vi "MPDSnC Engine.vi"(0 "Notifier Name":string, 11 "COM Port":string[](array[string])) -> ()   [LabVIEW 2016]
uses:
  AOTF Controls/AOTF Lines Lines Control.ctl
  AOTF Controls/AOTF Notifier Element.ctl
  AOTF Controls/AOTF Actions.ctl
  <vilib>/Instr/_visa.llb/VISA Configure Serial Port (Instr).vi
panel:
  in  "Line On/Off":bool
  in  "Laser Wavelength (nm)":string
  out "Write Response":string
  in  "Blank":bool
  in  "Quit":bool
  in  "Power":dbl(slide) scale=0.0..100.0
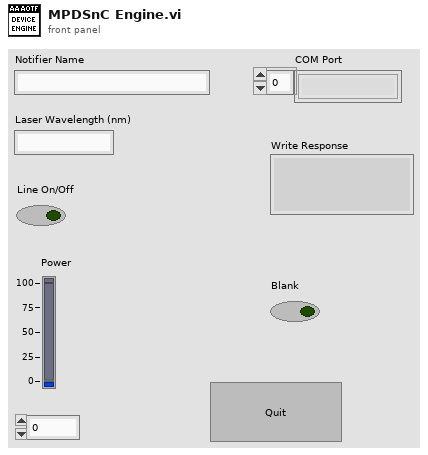
[diagram p1: front panel]
types:
  T1 = typedef "AOTF Notifier Element.ctl" = cluster{"AOTF Action":T2, "Laser Line":string, "Power (%)":dbl, "Beam Blank On/Off":bool, "Line On/Off":bool, "Error":errorcluster}
  T2 = typedef "AOTF Actions.ctl" = enum16{"Error Check", "Blank", "Line On/Off", "Set Power", "Status", "Quit"}
  T3 = typedef "AOTF Lines Lines Control.ctl" = cluster{"Wavelength":u16[], "AO Line":string[]}
  T4 = enum32{"Invalid", "Standard", "Closed", "Hidden", "Minimized", "Maximized"}
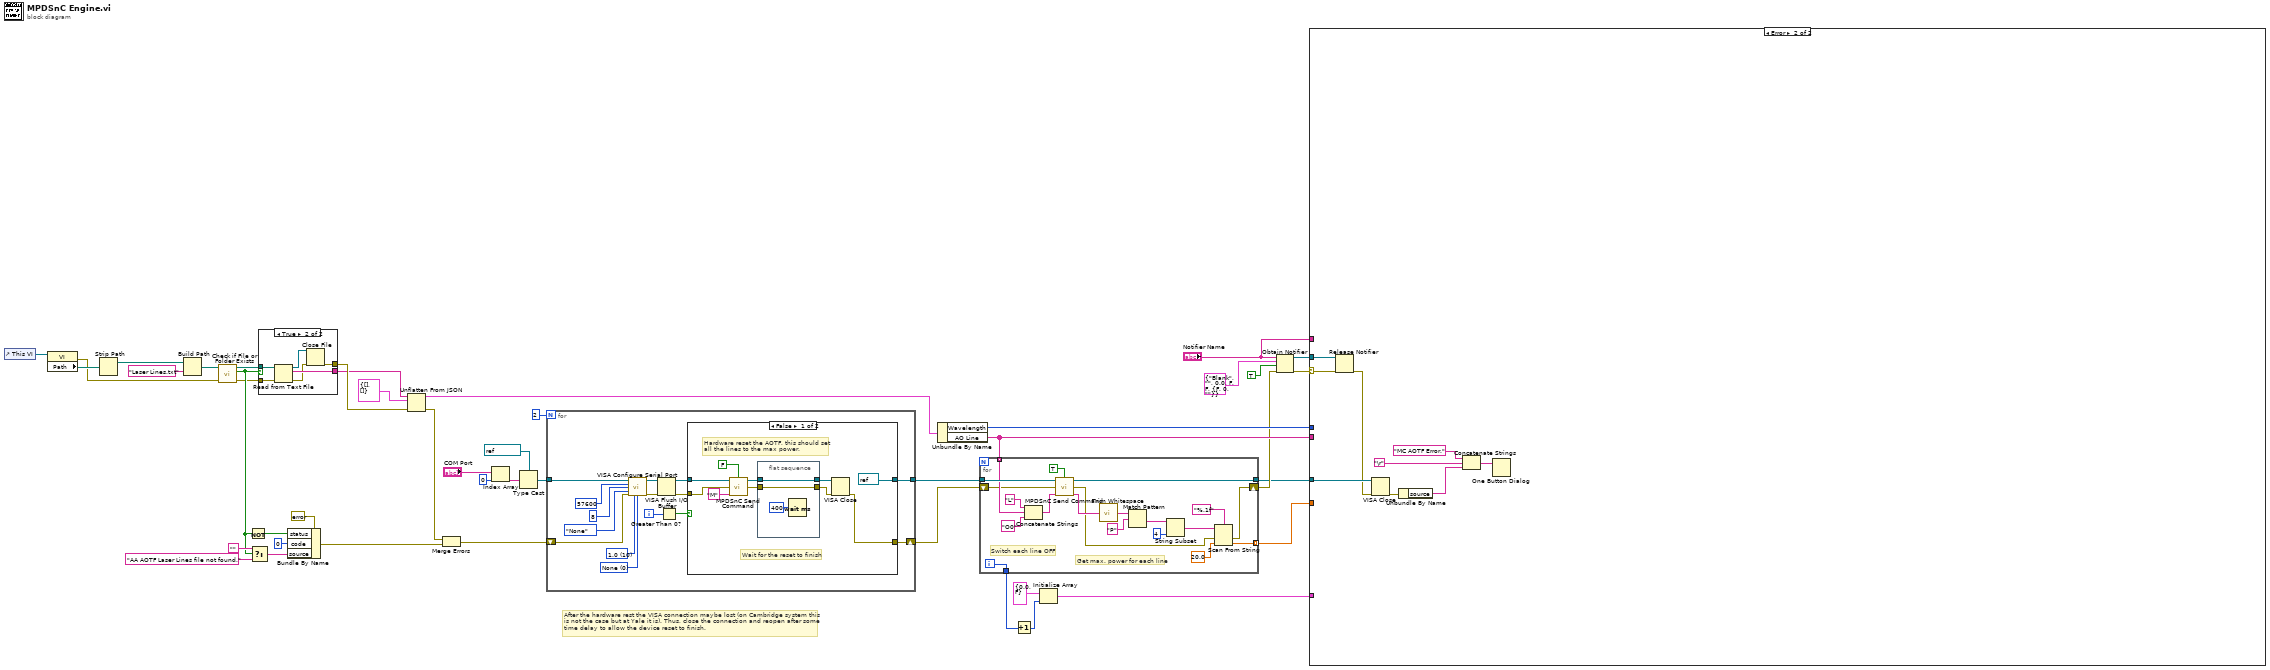
[diagram p0: block diagram]
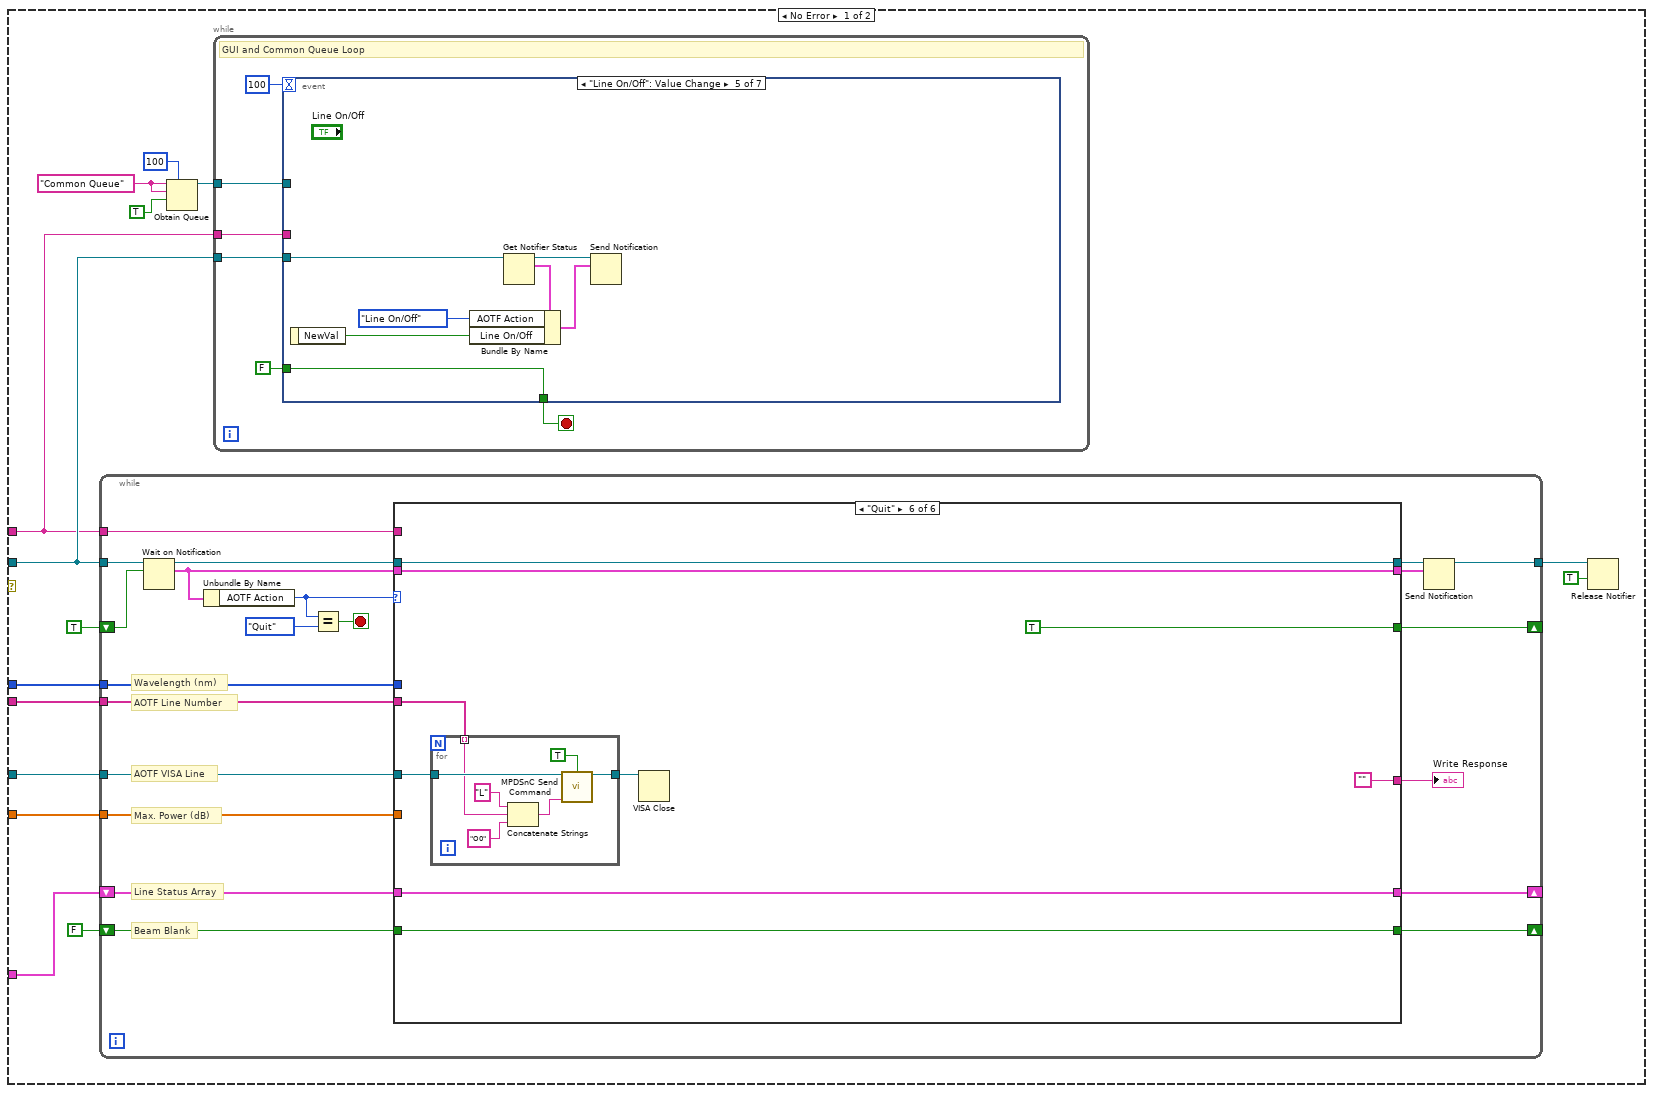
[diagram p3: hidden frame]
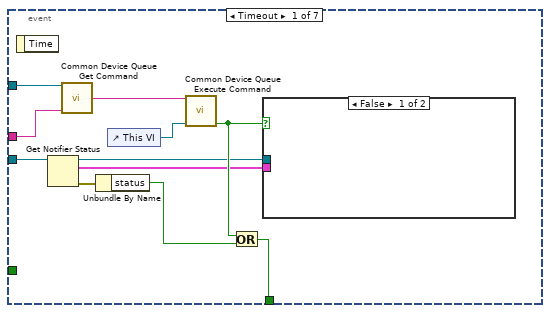
[diagram p4: hidden frame]
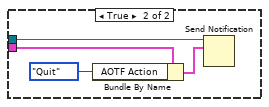
[diagram p5: hidden frame]
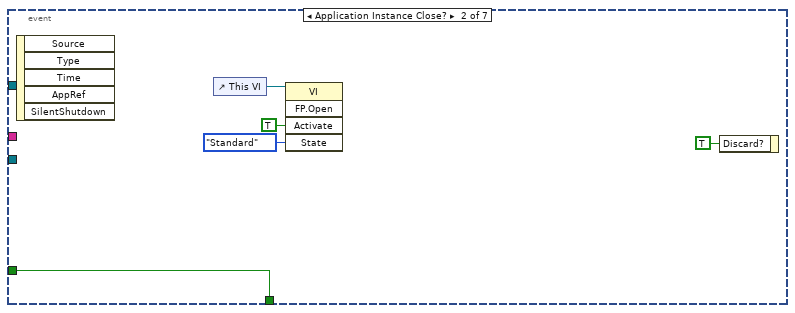
[diagram p6: hidden frame]
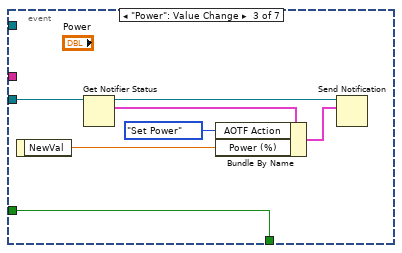
[diagram p7: hidden frame]
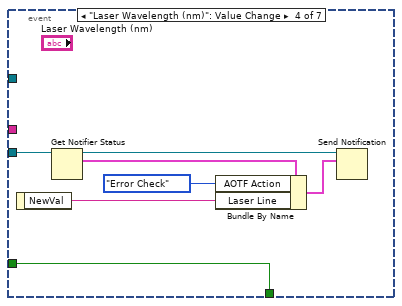
[diagram p8: hidden frame]
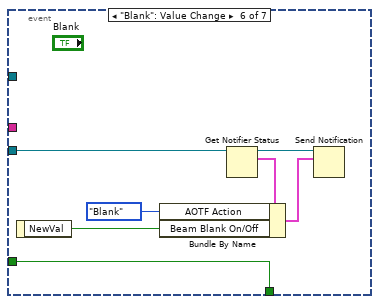
[diagram p9: hidden frame]
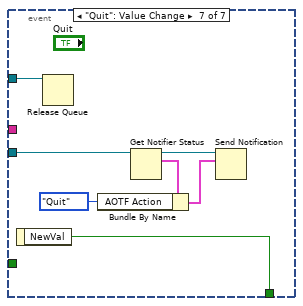
[diagram p10: hidden frame]
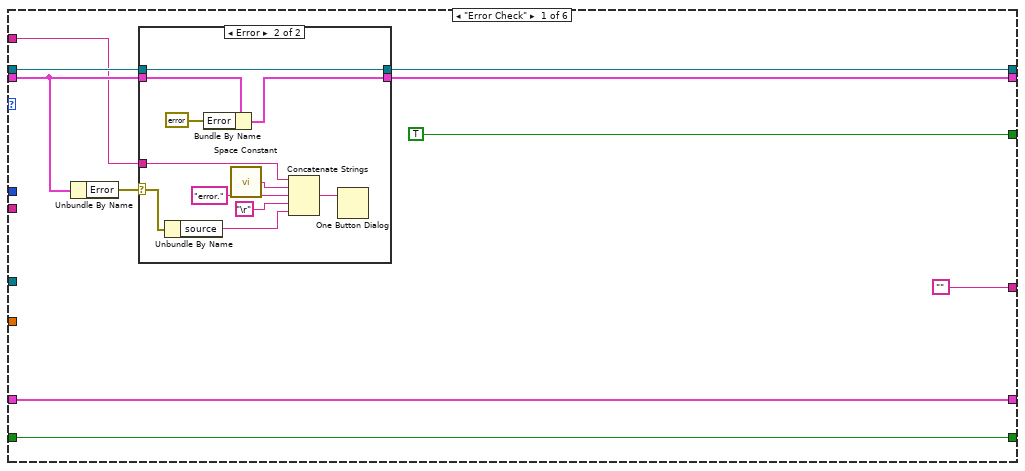
[diagram p11: hidden frame]
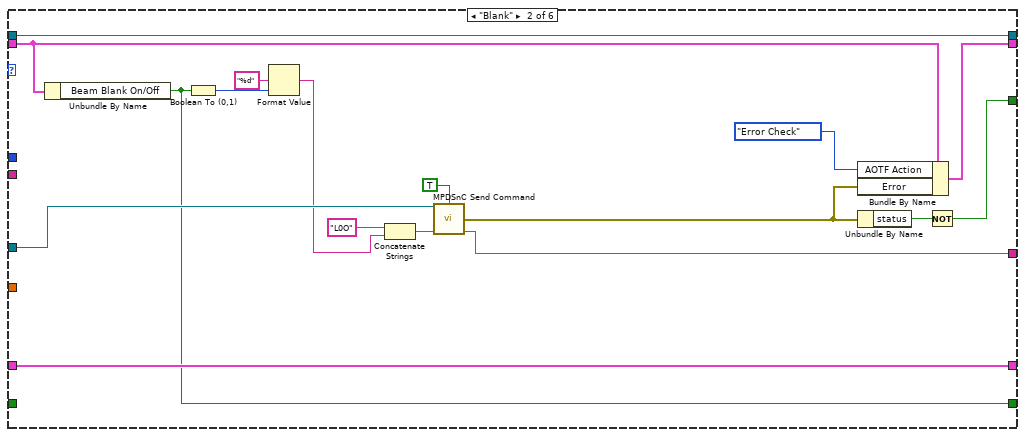
[diagram p13: hidden frame]
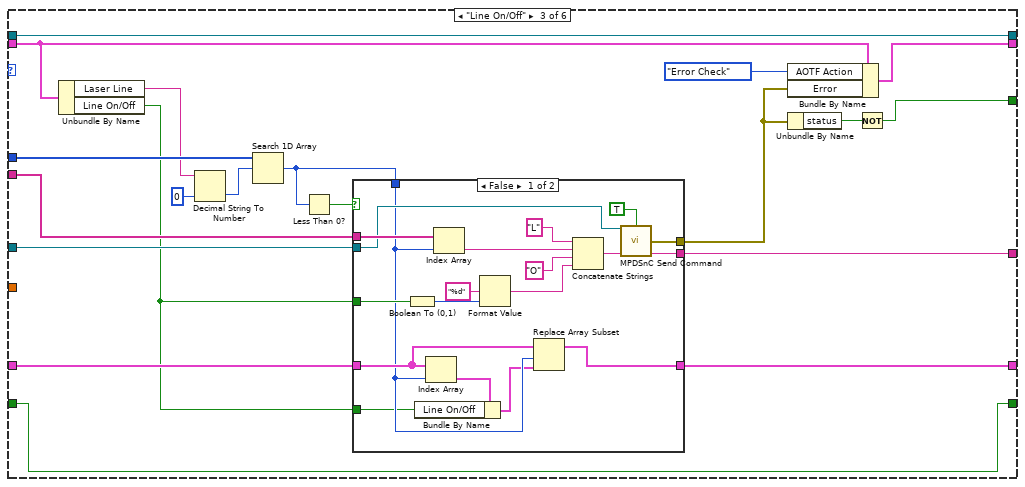
[diagram p14: hidden frame]
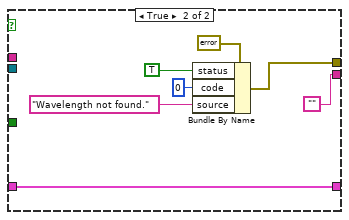
[diagram p15: hidden frame]
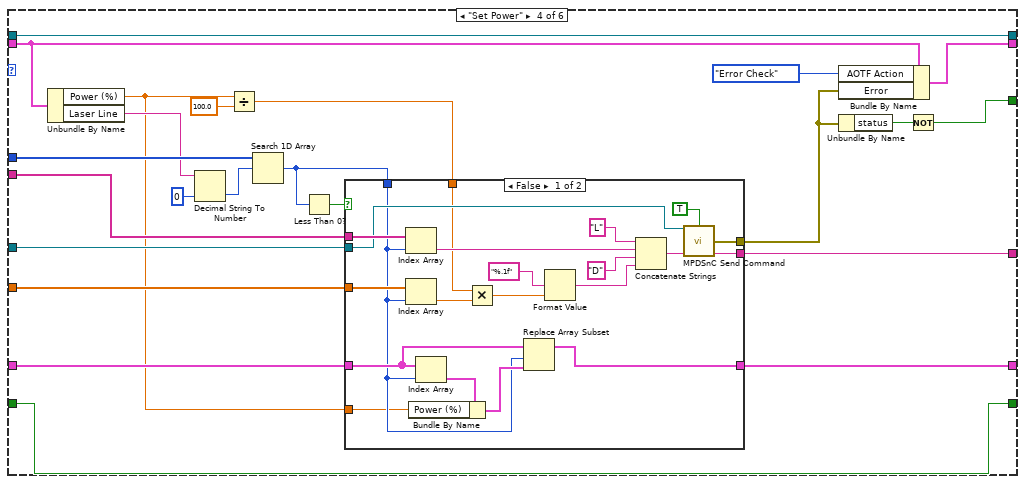
[diagram p16: hidden frame]
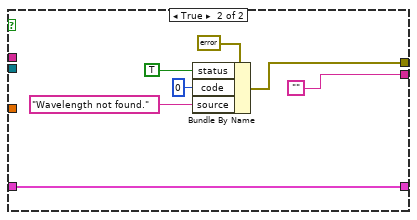
[diagram p17: hidden frame]
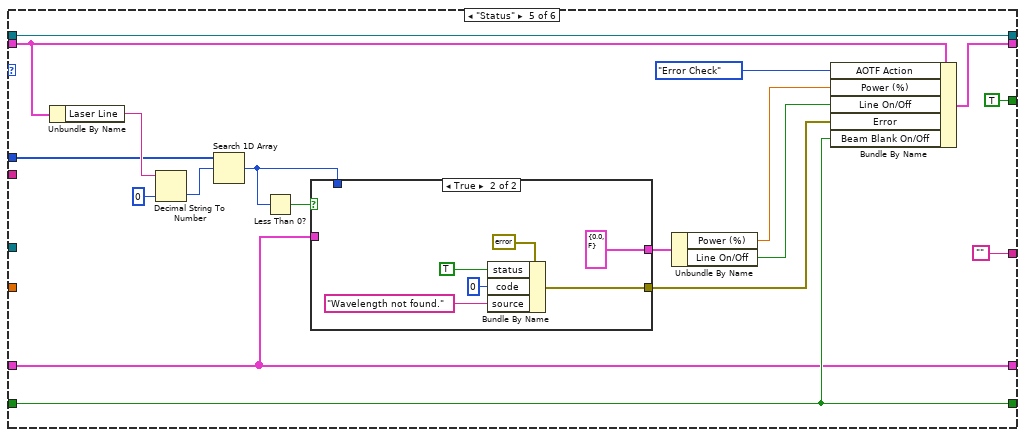
[diagram p18: hidden frame]
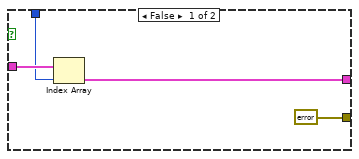
[diagram p19: hidden frame]
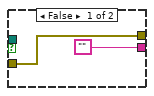
[diagram p20: hidden frame]
diagram:
  # "After the hardware rest the VISA connection maybe lost (on Cambridge system this\nis not the case but at Yale it is). Thus, close the connection and reopen after some\ntime delay to allow the device reset to finish."
  n1 = control-ref of="This VI"() -> (w44:refnum<vi>)
  n2 = property class="VI"(reference=w44) -> (error out=w31:errorcluster, "Path"=w43:path)  [unwired: 1 in, 1 out]
  n3 = Strip Path(path=w43) -> (stripped path=w42:path)  [unwired: 1 out]
  n4 = Build Path(base path=w42, name or relative path="Laser Lines.txt") -> (appended path=w40:path)
  n5 = call <vilib>:"Check if File or Folder Exists.vi"("error in (no error)"=w31, "path"=w40) -> ("error out"=w30:errorcluster, "file or folder exists?"=w33:bool, "dup path"=w32:path)  [unwired: 7 in]
  n6 = Not(x=w33) -> (.not. x?=w38:bool)
  n7 = Select(t="", s=w33, f="AA AOTF Laser Lines file not found." ("source")) -> (s? t:f=w34:string)
  n8 = case shown="True" w33 {
    tunnel: w32 -> [_ w52]
    tunnel: ["" w51] -> w26
    tunnel: w30 -> [w45 w49]
    tunnel: [w45 w47] -> w29
    frame False {
    }
    frame True {
      n9 = Read from Text File(file (use dialog)=w52, error in=w49) -> (refnum out=w50:refnum<file>, text=w51:string, error out=w48:errorcluster)  [unwired: 2 in, 1 out]
      n10 = Close File(refnum=w50, error in=w48) -> (error out=w47:errorcluster)  [unwired: 1 out]
    }
  }
  n11 = Bundle By Name(cluster=errorcluster {"status"=FALSE, "code"=0, "source"=""} ("Error"), "status"=w38, "code"=0, "source"=w34) -> (w27:errorcluster)
  n12 = Unflatten From JSON(JSON string=w26, type and defaults=T3 {"Wavelength"=[], "AO Line"=[]} ("Laser Lines"), error in (no error)=w29) -> (value=w24:T3, error out=w28:errorcluster)  [unwired: 4 in]
  n13 = Merge Errors(w28, w27) -> (w19:errorcluster)
  n14 = Index Array(array="COM Port", index=0) -> (element=w5:string)
  n15 = Type Cast(type=refnum<visa-resource-name> "COM6" ("reference"), x=w5) -> (*(type *) &x=w1:refnum<visa-resource-name>)
  n16 = for {
    N: 2 -> [_]
    tunnel: [w59] -> w21
    shift-right: [w57] -> w20
    shift-left: w19 -> [w56]
    tunnel: w1 -> [w53]
    i -> [w55]
    w67 = u16 0 items=["None", "XON/XOFF", "RTS/CTS", "XON/XOFF & RTS/CTS", "DTR/DSR", "XON/XOFF & DTR/DSR"] ("flow control (0:none)")
    w66 = u16 10 items=["1.0"=10, "1.5"=15, "2.0"=20] ("stop bits (10: 1 bit)")
    n17 = call-poly "VISA Configure Serial Port"("VISA resource name"=w53, "baud rate (9600)"=u32 57600, "data bits (8)"=u16 8, "parity (0:none)"=enum16{"None", "Odd", "Even", "Mark", "Space"}."None", "error in (no error)"=w56, "stop bits (10: 1 bit)"=w66, "flow control (0:none)"=w67) -> ("VISA resource name out"=w62:refnum<visa-resource-name>, "error out"=w61:errorcluster)  [unwired: 7 in]
    n18 = VISA Flush I/O Buffer(VISA resource name=w62, error in (no error)=w61) -> (VISA resource name out=w60:refnum<visa-resource-name>, error out=w58:errorcluster)  [unwired: 1 in]
    n19 = Greater Than 0?(x=w55) -> (x > 0?=w54:bool)
    n20 = case shown="False" w54 {
      tunnel: w60 -> [w77 w82]
      tunnel: [refnum<visa-resource-name> refnum ("VISA resource name") w82] -> w59
      tunnel: w58 -> [w76 w81]
      tunnel: [w69 w81] -> w57
      frame False {
        # "Wait for the reset to finish"
        # "Hardware reset the AOTF, this should set\nall the lines to the max power."
        n21 = call "MPDSnC Send Command.vi"("VISA Ref"=w77, "Wait for Reply?"=FALSE, "Error In"=w76, "Command"="M") -> ("VISA Ref Out"=w73:refnum<visa-resource-name>, "Error Out"=w72:errorcluster)  [unwired: 9 in, 1 out]
        n22 = flat-sequence {
          tunnel: [w80] -> w71
          tunnel: w73 -> [w80]
          tunnel: w72 -> [w78]
          tunnel: [w78] -> w70
          frame #0 {
            n23 = Wait (ms)(milliseconds to wait=u32 400) -> ()  [unwired: 1 out]
          }
        }
        n24 = VISA Close(VISA resource name=w71, error in (no error)=w70) -> (error out=w69:errorcluster)
      }
      frame True {
      }
    }
  }
  n25 = Unbundle By Name(w24) -> ("Wavelength"=w23:u16[], "AO Line"=w22:string[])
  n26 = for {
    tunnel: w21 -> [w101]
    tunnel: w22 -> [w99] mode=indexing
    tunnel: [w95] -> w11
    tunnel: [w88] -> w12 mode=indexing
    shift-right: [w84] -> w18
    shift-left: w20 -> [w86]
    tunnel: [w83] -> w9
    i -> [w83]
    # "Get max. power for each line"
    # "Switch each line OFF"
    n27 = Concatenate Strings("L", w99, "O0" ("string")) -> (w98:string)
    n28 = call "MPDSnC Send Command.vi"("VISA Ref"=w101, "Wait for Reply?"=TRUE, "Error In"=w86, "Command"=w98) -> ("VISA Ref Out"=w95:refnum<visa-resource-name>, "Error Out"=w85:errorcluster, "Response"=w96:string)  [unwired: 9 in]
    n29 = call <vilib>:"Trim Whitespace.vi"("string"=w96) -> ("trimmed string"=w94:string)  [unwired: 1 in]
    n30 = Match Pattern(string=w94, regular expression="P") -> (after substring=w92:string)  [unwired: 1 in, 3 out]
    n31 = String Subset(string=w92, length (rest)=4 ("length (rest)")) -> (substring=w90:string)  [unwired: 1 in]
    n32 = Scan From String(format string="%.1f", input string=w90, error in=w85, default 1=20.0 ("default value 1")) -> (error out=w84:errorcluster, output 1=w88:dbl)  [unwired: 1 in, 2 out]
  }
  n33 = Increment(x=w9) -> (x+1=w8:i32)
  n34 = Initialize Array(cluster{"Power (%)":dbl, "Line On/Off":bool} {"Power (%)"=0.0, "Line On/Off"=FALSE} ("Line Staus Cluster"), w8) -> (w7:cluster{"Power (%)":dbl, "Line On/Off":bool}[])
  n35 = Obtain Notifier(name (unnamed)="Notifier Name", notification data type=T1 {"AOTF Action"=enum."Blank", "Laser Line"="", "Power (%)"=0.0, "Beam Blank On/Off"=FALSE, "Line On/Off"=FALSE, "Error"={"status"=FALSE, "code"=0, "source"=""}} ("AOTFQueueCtrl"), create if not found? (T)=TRUE, error in (no error)=w18) -> (notifier out=w15:refnum<notifier>, error out=w14:errorcluster)  [unwired: 1 out]
  n36 = case shown="Error" w14 {
    selector: w14 -> [_ w388]
    tunnel: w15 -> [w113 w389]
    tunnel: "Notifier Name" -> [w109 _]
    tunnel: w23 -> [w108 _]
    tunnel: w22 -> [w107 _]
    tunnel: w12 -> [w106 _]
    tunnel: w11 -> [w105 w383]
    tunnel: w7 -> [w104 _]
    frame No Error {
      w117 = "Common Queue" ("Unique Notifier Name")
      n37 = while {
        tunnel: w113 -> [w199]
        shift-right: [w190] -> _
        shift-left: TRUE ("ignore previous (F)") -> [w198]
        tunnel: [w189] -> w111
        tunnel: w109 -> [w188]
        tunnel: w108 -> [w187]
        tunnel: w107 -> [w186]
        tunnel: w106 -> [w185]
        tunnel: w105 -> [w184]
        shift-right: [w179] -> _
        shift-left: w104 -> [w182]
        shift-right: [w180] -> _
        shift-left: FALSE -> [w181]
        stop <- w193 stop-if-true
        # "Wavelength (nm)"
        # "AOTF Line Number"
        # "Line Status Array"
        # "Beam Blank"
        # "AOTF VISA Line"
        # "Max. Power (dB)"
        n38 = Wait on Notification(notifier=w199, ignore previous (F)=w198) -> (notifier out=w197:refnum<notifier>, notification=w196:T1)  [unwired: 2 in, 2 out]
        n39 = Unbundle By Name(w196) -> ("AOTF Action"=w195:T2)
        n40 = Equal?(x=w195, y=AOTF_Actions."Quit") -> (x = y?=w193:bool)
        n41 = case shown="\"Quit\"" w195 {
          tunnel: w197 -> [w209 w239 w255 w308 w353 w373]
          tunnel: w196 -> [w207 w238 w257 w304 w348 w372]
          tunnel: [w205 w239 w255 w308 w353 w373] -> w192
          tunnel: [w204 w237 w256 w303 w344 w372] -> w191
          tunnel: [TRUE w234 w244 w302 TRUE TRUE] -> w190
          tunnel: w188 -> [w206 _ _ _ _ _]
          tunnel: w187 -> [_ _ w252 w299 w349 _]
          tunnel: w186 -> [_ _ w249 w295 _ w367]
          tunnel: w185 -> [_ _ _ w292 _ _]
          tunnel: w184 -> [_ w232 w248 w291 _ w366]
          tunnel: ["" w225 w246 w290 "" ""] -> w183
          tunnel: w182 -> [w201 w224 w243 w289 w337 w369]
          tunnel: w181 -> [w200 _ w241 w286 w338 w368]
          tunnel: [w200 w223 w241 w286 w338 w368] -> w180
          tunnel: [w201 w224 w242 w287 w337 w369] -> w179
          frame "Error Check" {
            n42 = Unbundle By Name(w207) -> ("Error"=w208:errorcluster)
            n43 = case shown="Error" w208 {
              selector: w208 -> [_ w215]
              tunnel: w207 -> [w210 w219]
              tunnel: [w211 w217] -> w205
              tunnel: w209 -> [w211 w217]
              tunnel: w206 -> [_ w214]
              tunnel: [w210 w216] -> w204
              frame No Error {
              }
              frame Error {
                n44 = Unbundle By Name(w215) -> ("source"=w213:string)
                n45 = Bundle By Name(cluster=w219, "Error"=errorcluster {"status"=FALSE, "code"=0, "source"=""}) -> (w216:T1)
                n46 = call <vilib>:"Space Constant.vi"() -> ("String"=w222:string)
                n47 = Concatenate Strings(w214, w222, "error." ("string"), "\r", w213) -> (w220:string)
                n48 = One Button Dialog(message=w220) -> ()  [unwired: 1 in, 1 out]
              }
            }
          }
          frame "Blank" {
            n49 = Unbundle By Name(w238) -> ("Beam Blank On/Off"=w223:bool)
            n50 = Boolean To (0,1)(Boolean=w223) -> (0, 1=w228:i16)
            n51 = Format Value(format string="%d", value (0)=w228) -> (output string=w226:string)  [unwired: 1 in]
            n52 = Concatenate Strings("L0O", w226) -> (w229:string)
            n53 = call "MPDSnC Send Command.vi"("VISA Ref"=w232, "Wait for Reply?"=TRUE, "Command"=w229) -> ("Error Out"=w233:errorcluster, "Response"=w225:string)  [unwired: 10 in, 1 out]
            n54 = Bundle By Name(cluster=w238, "AOTF Action"=AOTF_Actions."Error Check", "Error"=w233) -> (w237:T1)
            n55 = Unbundle By Name(w233) -> ("status"=w235:bool)
            n56 = Not(x=w235) -> (.not. x?=w234:bool)
          }
          frame "Line On/Off" {
            n57 = Unbundle By Name(w257) -> ("Laser Line"=w251:string, "Line On/Off"=w240:bool)
            n58 = Decimal String To Number(string=w251, default (0L)=u16 0 ("default (0 I32)")) -> (number=w254:u16)  [unwired: 1 in, 1 out]
            n59 = Search 1D Array(1D array=w252, element=w254) -> (index of element=w247:i32)  [unwired: 1 in]
            n60 = Less Than 0?(x=w247) -> (x < 0?=w250:bool)
            n61 = case shown="False" w250 {
              tunnel: w249 -> [w278 _]
              tunnel: [w273 w281] -> w245
              tunnel: w247 -> [w263 _]
              tunnel: w248 -> [w271 _]
              tunnel: [w270 ""] -> w246
              tunnel: w240 -> [w267 _]
              tunnel: w243 -> [w265 w279]
              tunnel: [w264 w279] -> w242
              tunnel: w240 -> [w260 _]
              frame False {
                n62 = Boolean To (0,1)(Boolean=w267) -> (0, 1=w269:i16)
                n63 = Index Array(array=w265, index=w263) -> (element=w262:cluster{"Power (%)":dbl, "Line On/Off":bool})
                n64 = Bundle By Name(cluster=w262, "Line On/Off"=w260) -> (w261:cluster{"Power (%)":dbl, "Line On/Off":bool})
                n65 = Index Array(array=w278, index=w263) -> (element=w277:string)
                n66 = Format Value(format string="%d", value (0)=w269) -> (output string=w266:string)  [unwired: 1 in]
                n67 = Replace Array Subset(array=w265, new element=w261, index=w263) -> (w264:cluster{"Power (%)":dbl, "Line On/Off":bool}[])
                n68 = Concatenate Strings("L", w277, "O", w266) -> (w274:string)
                n69 = call "MPDSnC Send Command.vi"("VISA Ref"=w271, "Wait for Reply?"=TRUE, "Command"=w274) -> ("Error Out"=w273:errorcluster, "Response"=w270:string)  [unwired: 10 in, 1 out]
              }
              frame True {
                n70 = Bundle By Name(cluster=errorcluster {"status"=FALSE, "code"=0, "source"=""} ("error out"), "status"=TRUE, "code"=0, "source"="Wavelength not found.") -> (w281:errorcluster)
              }
            }
            n71 = Bundle By Name(cluster=w257, "AOTF Action"=AOTF_Actions."Error Check", "Error"=w245) -> (w256:T1)
            n72 = Unbundle By Name(w245) -> ("status"=w258:bool)
            n73 = Not(x=w258) -> (.not. x?=w244:bool)
          }
          frame "Set Power" {
            n74 = Unbundle By Name(w304) -> ("Power (%)"=w288:dbl, "Laser Line"=w298:string)
            n75 = Decimal String To Number(string=w298, default (0L)=u16 0 ("default (0 I32)")) -> (number=w300:u16)  [unwired: 1 in, 1 out]
            n76 = Divide(x=w288, y=100.0) -> (x/y=w294:dbl)
            n77 = Search 1D Array(1D array=w299, element=w300) -> (index of element=w296:i32)  [unwired: 1 in]
            n78 = Less Than 0?(x=w296) -> (x < 0?=w297:bool)
            n79 = case shown="False" w297 {
              tunnel: w295 -> [w329 _]
              tunnel: [w322 w332] -> w293
              tunnel: w296 -> [w312 _]
              tunnel: w294 -> [w311 _]
              tunnel: w292 -> [w326 _]
              tunnel: w291 -> [w317 _]
              tunnel: [w316 ""] -> w290
              tunnel: w289 -> [w313 w330]
              tunnel: w288 -> [w310 _]
              tunnel: [w309 w330] -> w287
              frame False {
                n80 = Index Array(array=w329, index=w312) -> (element=w328:string)
                n81 = Index Array(array=w326, index=w312) -> (element=w324:dbl)
                n82 = Index Array(array=w313, index=w312) -> (element=w315:cluster{"Power (%)":dbl, "Line On/Off":bool})
                n83 = Bundle By Name(cluster=w315, "Power (%)"=w310) -> (w314:cluster{"Power (%)":dbl, "Line On/Off":bool})
                n84 = Multiply(x=w311, y=w324) -> (x*y=w319:dbl)
                n85 = Replace Array Subset(array=w313, new element=w314, index=w312) -> (w309:cluster{"Power (%)":dbl, "Line On/Off":bool}[])
                n86 = Format Value(format string="%.1f", value (0)=w319) -> (output string=w318:string)  [unwired: 1 in]
                n87 = Concatenate Strings("L", w328, "D", w318) -> (w323:string)
                n88 = call "MPDSnC Send Command.vi"("VISA Ref"=w317, "Wait for Reply?"=TRUE, "Command"=w323) -> ("Error Out"=w322:errorcluster, "Response"=w316:string)  [unwired: 10 in, 1 out]
              }
              frame True {
                n89 = Bundle By Name(cluster=errorcluster {"status"=FALSE, "code"=0, "source"=""} ("error out"), "status"=TRUE, "code"=0, "source"="Wavelength not found.") -> (w332:errorcluster)
              }
            }
            n90 = Bundle By Name(cluster=w304, "AOTF Action"=AOTF_Actions."Error Check", "Error"=w293) -> (w303:T1)
            n91 = Unbundle By Name(w293) -> ("status"=w305:bool)
            n92 = Not(x=w305) -> (.not. x?=w302:bool)
          }
          frame "Status" {
            n93 = Unbundle By Name(w348) -> ("Laser Line"=w350:string)
            n94 = Decimal String To Number(string=w350, default (0L)=u16 0 ("default (0 I32)")) -> (number=w351:u16)  [unwired: 1 in, 1 out]
            n95 = Search 1D Array(1D array=w349, element=w351) -> (index of element=w346:i32)  [unwired: 1 in]
            n96 = Less Than 0?(x=w346) -> (x < 0?=w347:bool)
            n97 = case shown="True" w347 {
              tunnel: w337 -> [w358 _]
              tunnel: [errorcluster {"status"=FALSE, "code"=0, "source"=""} ("error out") w360] -> w342
              tunnel: w346 -> [w357 _]
              tunnel: [w356 cluster{"Power (%)":dbl, "Line On/Off":bool} {"Power (%)"=0.0, "Line On/Off"=FALSE} ("Line Staus Cluster")] -> w341
              frame False {
                n98 = Index Array(array=w358, index=w357) -> (element=w356:cluster{"Power (%)":dbl, "Line On/Off":bool})
              }
              frame True {
                n99 = Bundle By Name(cluster=errorcluster {"status"=FALSE, "code"=0, "source"=""} ("error out"), "status"=TRUE, "code"=0, "source"="Wavelength not found.") -> (w360:errorcluster)
              }
            }
            n100 = Unbundle By Name(w341) -> ("Power (%)"=w340:dbl, "Line On/Off"=w339:bool)
            n101 = Bundle By Name(cluster=w348, "AOTF Action"=AOTF_Actions."Error Check", "Power (%)"=w340, "Line On/Off"=w339, "Error"=w342, "Beam Blank On/Off"=w338) -> (w344:T1)
          }
          frame "Quit" {
            n102 = for {
              tunnel: w366 -> [w379]
              tunnel: w367 -> [w377] mode=indexing
              tunnel: [w374] -> w365
              n103 = Concatenate Strings("L", w377, "O0" ("string")) -> (w376:string)
              n104 = call "MPDSnC Send Command.vi"("VISA Ref"=w379, "Wait for Reply?"=TRUE, "Command"=w376) -> ("VISA Ref Out"=w374:refnum<visa-resource-name>)  [unwired: 10 in, 2 out]
            }
            n105 = VISA Close(VISA resource name=w365) -> ()  [unwired: 1 in, 1 out]
          }
        }
        "Write Response" <- w183
        n106 = Send Notification(notification=w191, notifier=w192) -> (notifier out=w189:refnum<notifier>)  [unwired: 1 in, 1 out]
      }
      n107 = Obtain Queue(max queue size (-1, unlimited)=100, name (unnamed)=w117, element data type=w117, create if not found? (T)=TRUE) -> (queue out=w114:refnum<queue>)  [unwired: 1 in, 2 out]
      n108 = while {
        tunnel: w114 -> [w122]
        tunnel: w109 -> [w120]
        tunnel: w113 -> [w121]
        stop <- w119 stop-if-true
        # "GUI and Common Queue Loop"
        n109 = event shown="[4] \"Line On/Off\": Value Change" {
          selector: _ -> [_ _ _ _ _ _ _]
          dyn-events: _ -> [_ _ _ _ _ _ _]
          timeout: 100 -> [_ _ _ _ _ _ _]
          tunnel: w122 -> [w129 _ _ _ _ _ w178]
          tunnel: w121 -> [w125 _ w146 w153 w160 w170 w177]
          tunnel: w120 -> [w128 _ _ _ _ _ _]
          tunnel: [w127 w143 w150 w157 w164 w171 w175] -> w119
          tunnel: FALSE -> [_ w143 w150 w157 w164 w171 _]
          event Timeout {
            n110 = event-data() -> ()  [unwired: 1 in, 1 out]
            n111 = Get Notifier Status(notifier=w125) -> (notifier out=w124:refnum<notifier>, current notification=w126:T1, error out=w134:errorcluster)  [unwired: 1 in, 2 out]
            n112 = call "Common Device Queue Get Command.vi"("Common Queue"=w129, "Notifier Name"=w128) -> ("Command"=w133:string)  [unwired: 12 in, 1 out]
            n113 = Unbundle By Name(w134) -> ("status"=w131:bool)
            n114 = control-ref of="This VI"() -> (w132:refnum<vi>)
            n115 = call "Common Device Queue Execute Command.vi"("Common Command"=w133, "VI Refnum"=w132) -> ("Quit?"=w130:bool)  [unwired: 12 in, 1 out]
            n116 = Or(x=w130, y=w131) -> (x .or. y?=w127:bool)
            n117 = case shown="False" w130 {
              tunnel: w124 -> [_ w138]
              tunnel: w126 -> [_ w137]
              frame False {
              }
              frame True {
                n118 = Bundle By Name(cluster=w137, "AOTF Action"=AOTF_Actions."Quit") -> (w136:T1)
                n119 = Send Notification(notification=w136, notifier=w138) -> ()  [unwired: 1 in, 2 out]
              }
            }
          }
          event Application Instance Close? {
            n120 = event-data() -> ()  [unwired: 1 in, 5 out]
            n121 = control-ref of="This VI"() -> (w140:refnum<vi>)
            n122 = invoke class="VI" method="FP.Open"(reference=w140, "Activate"=TRUE ("Activate?"), "State"=T4."Standard") -> ()  [unwired: 2 in, 5 out]
            n123 = event-data("Discard?"=TRUE) -> ()  [unwired: 1 in, 1 out]
          }
          event "Power": Value Change {
            n124 = event-data() -> ("NewVal"=w148:dbl)  [unwired: 1 in]
            n125 = Get Notifier Status(notifier=w146) -> (notifier out=w144:refnum<notifier>, current notification=w145:T1)  [unwired: 1 in, 3 out]
            n126 = Bundle By Name(cluster=w145, "AOTF Action"=AOTF_Actions."Set Power", "Power (%)"=w148) -> (w147:T1)
            n127 = Send Notification(notification=w147, notifier=w144) -> ()  [unwired: 1 in, 2 out]
          }
          event "Laser Wavelength (nm)": Value Change {
            n128 = event-data() -> ("NewVal"=w155:string)  [unwired: 1 in]
            n129 = Get Notifier Status(notifier=w153) -> (notifier out=w151:refnum<notifier>, current notification=w152:T1)  [unwired: 1 in, 3 out]
            n130 = Bundle By Name(cluster=w152, "AOTF Action"=AOTF_Actions."Error Check", "Laser Line"=w155) -> (w154:T1)
            n131 = Send Notification(notification=w154, notifier=w151) -> ()  [unwired: 1 in, 2 out]
          }
          event "Line On/Off": Value Change {
            n132 = event-data() -> ("NewVal"=w159:bool)  [unwired: 1 in]
            n133 = Get Notifier Status(notifier=w160) -> (notifier out=w163:refnum<notifier>, current notification=w162:T1)  [unwired: 1 in, 3 out]
            n134 = Bundle By Name(cluster=w162, "AOTF Action"=AOTF_Actions."Line On/Off", "Line On/Off"=w159) -> (w158:T1)
            n135 = Send Notification(notification=w158, notifier=w163) -> ()  [unwired: 1 in, 2 out]
          }
          event "Blank": Value Change {
            n136 = event-data() -> ("NewVal"=w166:bool)  [unwired: 1 in]
            n137 = Get Notifier Status(notifier=w170) -> (notifier out=w169:refnum<notifier>, current notification=w168:T1)  [unwired: 1 in, 3 out]
            n138 = Bundle By Name(cluster=w168, "AOTF Action"=AOTF_Actions."Blank", "Beam Blank On/Off"=w166) -> (w165:T1)
            n139 = Send Notification(notification=w165, notifier=w169) -> ()  [unwired: 1 in, 2 out]
          }
          event "Quit": Value Change {
            n140 = event-data() -> ("NewVal"=w175:bool)  [unwired: 1 in]
            n141 = Release Queue(queue=w178) -> ()  [unwired: 2 in, 3 out]
            n142 = Get Notifier Status(notifier=w177) -> (notifier out=w176:refnum<notifier>, current notification=w174:T1)  [unwired: 1 in, 3 out]
            n143 = Bundle By Name(cluster=w174, "AOTF Action"=AOTF_Actions."Quit") -> (w172:T1)
            n144 = Send Notification(notification=w172, notifier=w176) -> ()  [unwired: 1 in, 2 out]
          }
        }
      }
      n145 = Release Notifier(notifier=w111, force destroy? (F)=TRUE) -> ()  [unwired: 1 in, 3 out]
    }
    frame Error {
      n146 = Release Notifier(notifier=w389, error in (no error)=w388) -> (error out=w382:errorcluster)  [unwired: 1 in, 2 out]
      n147 = VISA Close(VISA resource name=w383, error in (no error)=w382) -> (error out=w381:errorcluster)
      n148 = Unbundle By Name(w381) -> ("source"=w385:string)
      n149 = Concatenate Strings("MC AOTF Error.", "\r", w385) -> (w384:string)
      n150 = One Button Dialog(message=w384) -> ()  [unwired: 1 in, 1 out]
    }
  }
